vi "UNITEST MAIN v2.0.vi"() -> ()   [LabVIEW 2025] (continued)
        n1667 = Unbundle By Name(w2745) -> ("Main Screen.STOP"=w2752:refnum<vi>)
        n1668 = Unbundle By Name(w2745) -> ("Main Home Screen.GUI"=w2761:refnum<vi>)
        n1669 = property on="Property Node" class="TabCtl (strict)"(reference=w2757, "Value"=T16."HOME") -> (reference out=w2759:refnum<vi>, error out=w2758:errorcluster)  [unwired: 1 in]
        n1670 = property on="Property Node" class="TabCtl (strict)"(reference=w2761, "Value"=T15."Setup") -> (reference out=w2763:refnum<vi>, error out=w2762:errorcluster)  [unwired: 1 in]
        n1671 = property on="Property Node" class="Bool (strict)"(reference=w2753, "Visible"=TRUE ("Value"), "Value"=FALSE) -> (reference out=w2748:refnum<vi>, error out=w2754:errorcluster)  [unwired: 1 in]
        n1672 = property on="Property Node" class="Bool (strict)"(reference=w2752, "Value"=w2750, "Visible"=w2750) -> (reference out=w2747:refnum<vi>, error out=w2751:errorcluster)  [unwired: 1 in]
        n1673 = Close Reference(reference=w2763, error in (no error)=w2762) -> ()  [unwired: 1 out]
        n1674 = Close Reference(reference=w2759, error in (no error)=w2758) -> ()  [unwired: 1 out]
        n1675 = Close Reference(reference=w2748, error in (no error)=w2754) -> ()  [unwired: 1 out]
        n1676 = Close Reference(reference=w2747, error in (no error)=w2751) -> ()  [unwired: 1 out]
        n1677 = call "Reinitial Parameter After Test.vi"("error in (no error)"=w2765, "main ref"=w2745) -> ("error out"=w2746:errorcluster)  [unwired: 9 in]
      }
      frame "Start Test" {
        n1678 = Unbundle By Name(w2771) -> ("Environmental control.Acoustic Emission 3"=w2777:refnum<vi>)
        n1679 = property on="Property Node" class="Bool (strict)"(reference=w2777) -> (reference out=w2775:refnum<vi>, error out=w2776:errorcluster, "Value"=w2774:bool)  [unwired: 1 in]
        n1680 = Close Reference(reference=w2775, error in (no error)=w2776) -> ()  [unwired: 1 out]
        n1681 = case shown="True" w2774 {
          tunnel: w2773 -> [w2779 w2783]
          tunnel: [w2779 w2780] -> w2772
          tunnel: w2771 -> [_ w2781]
          frame False {
          }
          frame True {
            n1682 = call "Acq start.vi"("error in (no error)"=w2783, "Data Cluster"=w2781) -> ("error out"=w2782:errorcluster)  [unwired: 9 in]
            n1683 = call <vilib>:"Clear Errors.vi"("error in (no error)"=w2782) -> ("error out"=w2780:errorcluster)  [unwired: 5 in, 1 out]
          }
        }
        n1684 = call "Test Start Sequence.vi"("error in (no error)"=w2772, "Data Cluster"=w2771) -> ("error out"=w2778:errorcluster)  [unwired: 9 in]
      }
      frame "STOP" {
        n1685 = call "Test Stop.vi"("error in (no error)"=w2805, "Data Cluster"=w2784) -> ("error out"=w2785:errorcluster)  [unwired: 9 in]
        n1686 = Unbundle By Name(w2784) -> ("Main Screen.Load En"=w2804:refnum<vi>)
        n1687 = Unbundle By Name(w2784) -> ("Main Screen.CZ FF"=w2799:refnum<vi>)
        n1688 = Unbundle By Name(w2784) -> ("Main Screen.zFF"=w2796:refnum<vi>)
        n1689 = property on="Property Node" class="Bool (strict)"(reference=w2804, "DisabledEnum"=T31."Disabled and Grayed Out" ("Disabled")) -> (reference out=w2792:refnum<vi>, error out=w2803:errorcluster)  [unwired: 1 in]
        n1690 = property on="Property Node" class="Bool (strict)"(reference=w2799, "DisabledEnum"=T31."Disabled and Grayed Out" ("Disabled"), "Value"=FALSE ("Visible")) -> (reference out=w2798:refnum<vi>, error out=w2800:errorcluster)  [unwired: 1 in]
        n1691 = property on="Property Node" class="Bool (strict)"(reference=w2796, "DisabledEnum"=T31."Disabled and Grayed Out" ("Disabled"), "Value"=FALSE ("Visible")) -> (reference out=w2797:refnum<vi>, error out=w2795:errorcluster)  [unwired: 1 in]
        n1692 = Close Reference(reference=w2792, error in (no error)=w2803) -> ()  [unwired: 1 out]
        n1693 = Close Reference(reference=w2798, error in (no error)=w2800) -> ()  [unwired: 1 out]
        n1694 = Close Reference(reference=w2797, error in (no error)=w2795) -> ()  [unwired: 1 out]
        n1695 = Unbundle By Name(w2784) -> ("Environmental control.Acoustic Emission 3"=w2790:refnum<vi>)
        n1696 = property on="Property Node" class="Bool (strict)"(reference=w2790) -> (reference out=w2788:refnum<vi>, error out=w2789:errorcluster, "Value"=w2787:bool)  [unwired: 1 in]
        n1697 = Close Reference(reference=w2788, error in (no error)=w2789) -> ()  [unwired: 1 out]
        n1698 = case shown="False" w2787 {
          tunnel: w2785 -> [w2806 w2810]
          tunnel: [w2806 w2807] -> w2786
          tunnel: w2784 -> [_ w2808]
          frame False {
          }
          frame True {
            n1699 = call "Acq stop.vi"("error in (no error)"=w2810, "Data Cluster"=w2808) -> ("error out"=w2809:errorcluster)  [unwired: 9 in]
            n1700 = call <vilib>:"Clear Errors.vi"("error in (no error)"=w2809) -> ("error out"=w2807:errorcluster)  [unwired: 5 in, 1 out]
          }
        }
      }
      frame "PlaceModule" {
        n1701 = call "Place Module.vi"("error in (no error)"=w2813, "main ref"=w2811) -> ("error out"=w2812:errorcluster)  [unwired: 9 in]
      }
      frame "Stage Homing" {
        n1702 = call "HOMINING.vi"("error in (no error)"=w2816, "main ref"=w2814) -> ("error out"=w2815:errorcluster)  [unwired: 9 in]
      }
      frame "Clear 3" {
        n1703 = Unbundle By Name(w2818) -> ("Loading.Stribeck Table  For loading"=w2828:refnum<vi>)
        n1704 = Unbundle By Name(w2818) -> ("Loading.Clear 3"=w2819:refnum<vi>)
        n1705 = property on="Property Node" class="Bool (strict)"(reference=w2819, "Value"=FALSE) -> (reference out=w2821:refnum<vi>, error out=w2820:errorcluster)  [unwired: 1 in]
        n1706 = call "DATA ENCRYPT STRING FILE WRITE.vi"("error in (no error)"=w2824, "User Action"="User Pressed Clear  on Step Load Sequence", "main ref"=w2818) -> ("error out"=w2823:errorcluster)  [unwired: 6 in, 1 out]
        n1707 = property on="Property Node" class="Tbl (strict)"(reference=w2828, "Value"=string[][] []) -> (reference out=w2826:refnum<vi>, error out=w2827:errorcluster)  [unwired: 1 in]
        n1708 = Close Reference(reference=w2821, error in (no error)=w2820) -> ()  [unwired: 1 out]
        n1709 = Close Reference(reference=w2826, error in (no error)=w2827) -> ()  [unwired: 1 out]
      }
      frame "Set WTD" {
        n1710 = Unbundle By Name(w2829) -> ("Motion Module.Set WTD"=w2832:refnum<vi>)
        n1711 = property on="Property Node" class="Bool (strict)"(reference=w2832, "Value"=FALSE) -> (reference out=w2834:refnum<vi>, error out=w2833:errorcluster)  [unwired: 1 in]
        n1712 = call "DATA ENCRYPT STRING FILE WRITE.vi"("error in (no error)"=w2836, "User Action"="User Pressed  on Set Wear Track", "main ref"=w2829) -> ("error out"=w2835:errorcluster)  [unwired: 6 in, 1 out]
        n1713 = call "Sway wear trac set.vi"("error in (no error)"=w2835, "main ref"=w2829) -> ("error out"=w2830:errorcluster)  [unwired: 9 in]
        n1714 = Close Reference(reference=w2834, error in (no error)=w2833) -> ()  [unwired: 1 out]
      }
      frame "Import 2" {
        n1715 = call "File Dialog"("start path"=path "C:/LAB-IQ 150/User Defined Protocol", "error in"=w2845) -> ("selected path"=w2839:path, "cancelled"=w2842:bool, "error out"=w2844:errorcluster)  [unwired: 10 in, 1 out]
        n1716 = call <vilib>:"Clear Errors.vi"("error in (no error)"=w2844) -> ("error out"=w2841:errorcluster)  [unwired: 5 in, 1 out]
        n1717 = case shown="False" w2842 {
          tunnel: w2841 -> [w2855 w2856]
          tunnel: [w2847 w2856] -> w2840
          tunnel: w2839 -> [w2854 _]
          tunnel: w2838 -> [w2849 _]
          frame False {
            n1718 = call-poly <vilib>:"Read Delimited Spreadsheet.vi"("file path (dialog if empty)"=w2854, "error in (no error)"=w2855, "delimiter (\\t)"=":" ("delimiter (\\t)")) -> ("all rows"=w2846:string[][], "error out"=w2848:errorcluster)  [unwired: 7 in, 4 out]
            n1719 = Unbundle By Name(w2849) -> ("Motion Module.StepTable For Speed"=w2852:refnum<vi>)
            n1720 = property on="Property Node" class="Tbl (strict)"(reference=w2852, error in=w2848, "Value"=w2846) -> (reference out=w2850:refnum<vi>, error out=w2851:errorcluster)
            n1721 = Close Reference(reference=w2850, error in (no error)=w2851) -> (error out=w2847:errorcluster)
          }
          frame True {
          }
        }
      }
      frame "Save 2" {
        n1722 = Unbundle By Name(w2860) -> ("Motion Module.StepTable For Speed"=w2875:refnum<vi>)
        n1723 = property on="Property Node" class="Tbl (strict)"(reference=w2875) -> (reference out=w2873:refnum<vi>, error out=w2874:errorcluster, "Value"=w2871:string[][])  [unwired: 1 in]
        n1724 = call "File Dialog2"("start path"=path "C:/LAB-IQ 150/User Defined Protocol", "error in"=w2865) -> ("selected path"=w2868:path, "error out"=w2867:errorcluster)  [unwired: 10 in, 2 out]
        n1725 = call <vilib>:"Clear Errors.vi"("error in (no error)"=w2867) -> ("error out"=w2866:errorcluster)  [unwired: 5 in, 1 out]
        n1726 = Close Reference(reference=w2873, error in (no error)=w2874) -> ()  [unwired: 1 out]
        n1727 = call-poly <vilib>:"Write Delimited Spreadsheet.vi"("file path (dialog if empty)"=w2868, "2D data"=w2871, "append to file? (new file:F)"=TRUE, "error in (no error)"=w2866, "delimiter (\\t)"=":" ("delimiter (\\t)")) -> ("error out"=w2864:errorcluster)  [unwired: 9 in, 1 out]
        n1728 = call <vilib>:"Clear Errors.vi"("error in (no error)"=w2864) -> ("error out"=w2859:errorcluster)  [unwired: 5 in, 1 out]
        n1729 = Unbundle By Name(w2860) -> ("Motion Module.Save 2"=w2861:refnum<vi>)
        n1730 = property on="Property Node" class="Bool (strict)"(reference=w2861, error in=w2859, "Value"=FALSE) -> (reference out=w2863:refnum<vi>, error out=w2862:errorcluster)
        n1731 = Close Reference(reference=w2863, error in (no error)=w2862) -> (error out=w2858:errorcluster)
      }
      frame "Calculate Rotary" {
        n1732 = call "STEP LOAD MM_SEC AND RPM CONVERSION.vi"("error in (no error)"=w2879, "Data Cluster"=w2877) -> ("error out"=w2878:errorcluster)  [unwired: 9 in]
        n1733 = local write "calculate rotary"(FALSE) -> ()
      }
      frame "Clear List" {
        n1734 = Unbundle By Name(w2881) -> ("Environmental control.Sensors Picked"=w2888:refnum<vi>)
        n1735 = Unbundle By Name(w2881) -> ("Environmental control.Clear List"=w2882:refnum<vi>)
        n1736 = property on="Property Node" class="Bool (strict)"(reference=w2882, "Value"=FALSE) -> (reference out=w2884:refnum<vi>, error out=w2883:errorcluster)  [unwired: 1 in]
        n1737 = property on="Property Node" class="Str"(reference=w2888, "Value"="") -> (reference out=w2886:refnum<vi>, error out=w2887:errorcluster)  [unwired: 1 in]
        n1738 = Close Reference(reference=w2884, error in (no error)=w2883) -> ()  [unwired: 1 out]
        n1739 = Close Reference(reference=w2886, error in (no error)=w2887) -> ()  [unwired: 1 out]
      }
      frame "ClrLog" {
        n1740 = Unbundle By Name(w2891) -> ("Main Screen.ClrLog"=w2892:refnum<vi>)
        n1741 = Unbundle By Name(w2891) -> ("Main Screen.Trip Log"=w2898:refnum<vi>)
        n1742 = property on="Property Node" class="Bool (strict)"(reference=w2892, "Value"=FALSE) -> (reference out=w2894:refnum<vi>, error out=w2893:errorcluster)  [unwired: 1 in]
        n1743 = property on="Property Node" class="Str"(reference=w2898, "Value"="") -> (reference out=w2896:refnum<vi>, error out=w2897:errorcluster)  [unwired: 1 in]
        n1744 = Close Reference(reference=w2894, error in (no error)=w2893) -> ()  [unwired: 1 out]
        n1745 = Close Reference(reference=w2896, error in (no error)=w2897) -> ()  [unwired: 1 out]
      }
      frame "Add to list" {
        n1746 = Unbundle By Name(w2900) -> ("Environmental control.Sensors Picked"=w2906:refnum<vi>)
        n1747 = property on="Property Node" class="Str"(reference=w2906, error in=w2901, "Value"="") -> (reference out=w2904:refnum<vi>, error out=w2905:errorcluster)
        n1748 = Close Reference(reference=w2904, error in (no error)=w2905) -> (error out=w2902:errorcluster)
        n1749 = call "Add  to List Loop.vi"("error in (no error)"=w2902, "Data Cluster"=w2900) -> ("error out"=w2908:errorcluster)  [unwired: 9 in]
        n1750 = Unbundle By Name(w2900) -> ("Environmental control.Add to list"=w2910:refnum<vi>)
        n1751 = property on="Property Node" class="Bool (strict)"(reference=w2910, error in=w2908, "Value"=FALSE) -> (reference out=w2912:refnum<vi>, error out=w2911:errorcluster)
        n1752 = Close Reference(reference=w2912, error in (no error)=w2911) -> (error out=w2907:errorcluster)
      }
      frame "Disable Axis Jog Soft Limits" {
        n1753 = call "DATA ENCRYPT STRING FILE WRITE.vi"("error in (no error)"=w2916, "User Action"="User Pressed Disable Axis Jog Soft Limits in Main Screen", "main ref"=w2914) -> ("error out"=w2915:errorcluster)  [unwired: 6 in, 1 out]
      }
      frame "Home Service" {
        n1754 = Unbundle By Name(w2918) -> ("Main Home Screen.MainPage"=w2924:refnum<vi>)
        n1755 = Unbundle By Name(w2918) -> ("Main Home Screen.GUI"=w2922:refnum<vi>)
        n1756 = local write "Home Service"(FALSE ("Home Service")) -> ()
        n1757 = property on="Property Node" class="TabCtl (strict)"(reference=w2924, "Value"=T16."HOME") -> (reference out=w2926:refnum<vi>, error out=w2925:errorcluster)  [unwired: 1 in]
        n1758 = property on="Property Node" class="TabCtl (strict)"(reference=w2922, "Value"=T15."Setup") -> (reference out=w2920:refnum<vi>, error out=w2921:errorcluster)  [unwired: 1 in]
        n1759 = Close Reference(reference=w2926, error in (no error)=w2925) -> ()  [unwired: 1 out]
        n1760 = Close Reference(reference=w2920, error in (no error)=w2921) -> ()  [unwired: 1 out]
        n1761 = call "DATA ENCRYPT STRING FILE WRITE.vi"("error in (no error)"=w2929, "User Action"="User Pressed Home Service from Service Screen", "main ref"=w2918) -> ("error out"=w2928:errorcluster)  [unwired: 6 in, 1 out]
      }
      frame "Analysis Home" {
        n1762 = Unbundle By Name(w2931) -> ("Main Screen.Main Screen Tab"=w2934:refnum<vi>)
        n1763 = Unbundle By Name(w2931) -> ("Main Home Screen.MainPage"=w2941:refnum<vi>)
        n1764 = Unbundle By Name(w2931) -> ("Main Home Screen.GUI"=w2939:refnum<vi>)
        n1765 = local write "Analysis Home new"(FALSE ("Analysis Home new")) -> ()
        n1766 = property on="Property Node" class="TabCtl (strict)"(reference=w2934, "Value"=T19."  Acquire  ") -> (reference out=w2932:refnum<vi>, error out=w2933:errorcluster)  [unwired: 1 in]
        n1767 = property on="Property Node" class="TabCtl (strict)"(reference=w2941, "Value"=T16."HOME") -> (reference out=w2943:refnum<vi>, error out=w2942:errorcluster)  [unwired: 1 in]
        n1768 = property on="Property Node" class="TabCtl (strict)"(reference=w2939, "Value"=T15."Setup") -> (reference out=w2937:refnum<vi>, error out=w2938:errorcluster)  [unwired: 1 in]
        n1769 = Close Reference(reference=w2932, error in (no error)=w2933) -> ()  [unwired: 1 out]
        n1770 = Close Reference(reference=w2943, error in (no error)=w2942) -> ()  [unwired: 1 out]
        n1771 = Close Reference(reference=w2937, error in (no error)=w2938) -> ()  [unwired: 1 out]
        n1772 = call "DATA ENCRYPT STRING FILE WRITE.vi"("error in (no error)"=w2946, "User Action"="User Pressed Home from AnalysisScreen", "main ref"=w2931) -> ("error out"=w2945:errorcluster)  [unwired: 6 in, 1 out]
      }
      frame "Post Analysis" {
        n1773 = Unbundle By Name(w2949) -> ("Main Screen.Main Screen Tab"=w2952:refnum<vi>)
        n1774 = Unbundle By Name(w2949) -> ("Main Home Screen.MainPage"=w2958:refnum<vi>)
        n1775 = Unbundle By Name(w2949) -> ("Main Home Screen.GUI"=w2956:refnum<vi>)
        n1776 = property on="Property Node" class="TabCtl (strict)"(reference=w2952, "Value"=T19."Compare Files Rot") -> (reference out=w2950:refnum<vi>, error out=w2951:errorcluster)  [unwired: 1 in]
        n1777 = property on="Property Node" class="TabCtl (strict)"(reference=w2958, "Value"=T16."HOME") -> (reference out=w2960:refnum<vi>, error out=w2959:errorcluster)  [unwired: 1 in]
        n1778 = property on="Property Node" class="TabCtl (strict)"(reference=w2956, "Value"=T15."Begin") -> (reference out=w2954:refnum<vi>, error out=w2955:errorcluster)  [unwired: 1 in]
        n1779 = local write "Post Analysis"(FALSE ("Post Analysis")) -> ()
        n1780 = Close Reference(reference=w2950, error in (no error)=w2951) -> ()  [unwired: 1 out]
        n1781 = Close Reference(reference=w2960, error in (no error)=w2959) -> ()  [unwired: 1 out]
        n1782 = Close Reference(reference=w2954, error in (no error)=w2955) -> ()  [unwired: 1 out]
        n1783 = call "DATA ENCRYPT STRING FILE WRITE.vi"("error in (no error)"=w2963, "User Action"="User Pressed Post Analysis ", "main ref"=w2949) -> ("error out"=w2962:errorcluster)  [unwired: 6 in, 1 out]
      }
      frame "Edit Gain Constants" {
        n1784 = Unbundle By Name(w2965) -> ("About Screen.Heave and Surge COM Port:"=w2995:refnum<vi>)
        n1785 = Unbundle By Name(w2965) -> ("About Screen.Edit Gain Constants"=w2975:refnum<vi>)
        n1786 = Unbundle By Name(w2965) -> ("About Screen.Sway COM Port:"=w2992:refnum<vi>)
        n1787 = Unbundle By Name(w2965) -> ("About Screen.Ramp Port:"=w2969:refnum<vi>)
        n1788 = Unbundle By Name(w2965) -> ("About Screen.Temp Modbus:"=w2989:refnum<vi>)
        n1789 = Unbundle By Name(w2965) -> ("About Screen.Humidity Port:"=w2988:refnum<vi>)
        n1790 = Unbundle By Name(w2965) -> ("About Screen.Password"=w2983:refnum<vi>)
        n1791 = Unbundle By Name(w2965) -> ("About Screen.ECR Port:"=w2968:refnum<vi>)
        n1792 = property on="Property Node" class="VISAName"(reference=w2969, "DisabledEnum"=T31."Enabled" ("Disabled")) -> (reference out=w2971:refnum<vi>, error out=w2970:errorcluster)  [unwired: 1 in]
        n1793 = property on="Property Node" class="Bool (strict)"(reference=w2975, "Value"=FALSE) -> (reference out=w2976:refnum<vi>, error out=w2974:errorcluster)  [unwired: 1 in]
        n1794 = property on="Property Node" class="VISAName"(reference=w2968, "DisabledEnum"=T31."Enabled" ("Disabled")) -> (reference out=w2964:refnum<vi>, error out=w2967:errorcluster)  [unwired: 1 in]
        n1795 = property on="Property Node" class="VISAName"(reference=w2995, "DisabledEnum"=T31."Enabled" ("Disabled")) -> (reference out=w2996:refnum<vi>, error out=w2994:errorcluster)  [unwired: 1 in]
        n1796 = property on="Property Node" class="VISAName"(reference=w2992, "DisabledEnum"=T31."Enabled" ("Disabled")) -> (reference out=w2993:refnum<vi>, error out=w2991:errorcluster)  [unwired: 1 in]
        n1797 = property on="Property Node" class="VISAName"(reference=w2989, "DisabledEnum"=T31."Enabled" ("Disabled")) -> (reference out=w2977:refnum<vi>, error out=w2990:errorcluster)  [unwired: 1 in]
        n1798 = property on="Property Node" class="VISAName"(reference=w2988, "DisabledEnum"=T31."Enabled" ("Disabled")) -> (reference out=w2986:refnum<vi>, error out=w2987:errorcluster)  [unwired: 1 in]
        n1799 = property on="Property Node" class="Str"(reference=w2983, "Visible"=FALSE) -> (reference out=w2985:refnum<vi>, error out=w2984:errorcluster)  [unwired: 1 in]
        n1800 = Close Reference(reference=w2971, error in (no error)=w2970) -> ()  [unwired: 1 out]
        n1801 = Close Reference(reference=w2985, error in (no error)=w2984) -> ()  [unwired: 1 out]
        n1802 = Close Reference(reference=w2964, error in (no error)=w2967) -> ()  [unwired: 1 out]
        n1803 = Close Reference(reference=w2976, error in (no error)=w2974) -> ()  [unwired: 1 out]
        n1804 = Close Reference(reference=w2996, error in (no error)=w2994) -> ()  [unwired: 1 out]
        n1805 = Close Reference(reference=w2993, error in (no error)=w2991) -> ()  [unwired: 1 out]
        n1806 = Close Reference(reference=w2977, error in (no error)=w2990) -> ()  [unwired: 1 out]
        n1807 = Close Reference(reference=w2986, error in (no error)=w2987) -> ()  [unwired: 1 out]
        n1808 = call "DATA ENCRYPT STRING FILE WRITE.vi"("error in (no error)"=w2999, "User Action"="User Pressed Home Service from Service Screen", "main ref"=w2965) -> ("error out"=w2998:errorcluster)  [unwired: 6 in, 1 out]
      }
      frame "Advanced Setting" {
        n1809 = Unbundle By Name(w3001) -> ("About Screen.Advanced Setting"=w3003:refnum<vi>)
        n1810 = property on="Property Node" class="Bool (strict)"(reference=w3003) -> (reference out=w3004:refnum<vi>, error out=w3002:errorcluster, "Value"=w3000:bool)  [unwired: 1 in]
        n1811 = Close Reference(reference=w3004, error in (no error)=w3002) -> ()  [unwired: 1 out]
        n1812 = case shown="True" w3000 {
          tunnel: w3001 -> [w3009 w3034]
          frame True {
            n1813 = Unbundle By Name(w3009) -> ("About Screen.Heave and Surge COM Port:"=w3031:refnum<vi>)
            n1814 = Unbundle By Name(w3009) -> ("About Screen.Edit Gain Constants"=w3011:refnum<vi>)
            n1815 = Unbundle By Name(w3009) -> ("About Screen.Sway COM Port:"=w3028:refnum<vi>)
            n1816 = Unbundle By Name(w3009) -> ("About Screen.Temp Modbus:"=w3025:refnum<vi>)
            n1817 = Unbundle By Name(w3009) -> ("About Screen.Humidity Port:"=w3024:refnum<vi>)
            n1818 = Unbundle By Name(w3009) -> ("About Screen.Password"=w3019:refnum<vi>)
            n1819 = property on="Property Node" class="Bool (strict)"(reference=w3011, "Value"=FALSE) -> (reference out=w3012:refnum<vi>, error out=w3010:errorcluster)  [unwired: 1 in]
            n1820 = property on="Property Node" class="VISAName"(reference=w3031, "DisabledEnum"=T31."Disabled and Grayed Out" ("Disabled")) -> (reference out=w3032:refnum<vi>, error out=w3030:errorcluster)  [unwired: 1 in]
            n1821 = property on="Property Node" class="VISAName"(reference=w3028, "DisabledEnum"=T31."Disabled and Grayed Out" ("Disabled")) -> (reference out=w3029:refnum<vi>, error out=w3027:errorcluster)  [unwired: 1 in]
            n1822 = property on="Property Node" class="VISAName"(reference=w3025, "DisabledEnum"=T31."Disabled and Grayed Out" ("Disabled")) -> (reference out=w3013:refnum<vi>, error out=w3026:errorcluster)  [unwired: 1 in]
            n1823 = property on="Property Node" class="VISAName"(reference=w3024, "DisabledEnum"=T31."Disabled and Grayed Out" ("Disabled")) -> (reference out=w3022:refnum<vi>, error out=w3023:errorcluster)  [unwired: 1 in]
            n1824 = property on="Property Node" class="Str"(reference=w3019, "Visible"=TRUE) -> (reference out=w3021:refnum<vi>, error out=w3020:errorcluster)  [unwired: 1 in]
            n1825 = Close Reference(reference=w3012, error in (no error)=w3010) -> ()  [unwired: 1 out]
            n1826 = Close Reference(reference=w3032, error in (no error)=w3030) -> ()  [unwired: 1 out]
            n1827 = Close Reference(reference=w3029, error in (no error)=w3027) -> ()  [unwired: 1 out]
            n1828 = Close Reference(reference=w3013, error in (no error)=w3026) -> ()  [unwired: 1 out]
            n1829 = Close Reference(reference=w3022, error in (no error)=w3023) -> ()  [unwired: 1 out]
            n1830 = Close Reference(reference=w3021, error in (no error)=w3020) -> ()  [unwired: 1 out]
          }
          frame False {
            n1831 = Unbundle By Name(w3034) -> ("About Screen.Heave and Surge COM Port:"=w3056:refnum<vi>)
            n1832 = Unbundle By Name(w3034) -> ("About Screen.Edit Gain Constants"=w3036:refnum<vi>)
            n1833 = Unbundle By Name(w3034) -> ("About Screen.Sway COM Port:"=w3053:refnum<vi>)
            n1834 = Unbundle By Name(w3034) -> ("About Screen.Temp Modbus:"=w3050:refnum<vi>)
            n1835 = Unbundle By Name(w3034) -> ("About Screen.Humidity Port:"=w3049:refnum<vi>)
            n1836 = Unbundle By Name(w3034) -> ("About Screen.Password"=w3044:refnum<vi>)
            n1837 = property on="Property Node" class="Bool (strict)"(reference=w3036, "Value"=FALSE) -> (reference out=w3037:refnum<vi>, error out=w3035:errorcluster)  [unwired: 1 in]
            n1838 = property on="Property Node" class="VISAName"(reference=w3056, "DisabledEnum"=T31."Disabled and Grayed Out" ("Disabled")) -> (reference out=w3057:refnum<vi>, error out=w3055:errorcluster)  [unwired: 1 in]
            n1839 = property on="Property Node" class="VISAName"(reference=w3053, "DisabledEnum"=T31."Disabled and Grayed Out" ("Disabled")) -> (reference out=w3054:refnum<vi>, error out=w3052:errorcluster)  [unwired: 1 in]
            n1840 = property on="Property Node" class="VISAName"(reference=w3050, "DisabledEnum"=T31."Disabled and Grayed Out" ("Disabled")) -> (reference out=w3038:refnum<vi>, error out=w3051:errorcluster)  [unwired: 1 in]
            n1841 = property on="Property Node" class="VISAName"(reference=w3049, "DisabledEnum"=T31."Disabled and Grayed Out" ("Disabled")) -> (reference out=w3047:refnum<vi>, error out=w3048:errorcluster)  [unwired: 1 in]
            n1842 = property on="Property Node" class="Str"(reference=w3044, "Visible"=FALSE) -> (reference out=w3046:refnum<vi>, error out=w3045:errorcluster)  [unwired: 1 in]
            n1843 = Close Reference(reference=w3037, error in (no error)=w3035) -> ()  [unwired: 1 out]
            n1844 = Close Reference(reference=w3057, error in (no error)=w3055) -> ()  [unwired: 1 out]
            n1845 = Close Reference(reference=w3054, error in (no error)=w3052) -> ()  [unwired: 1 out]
            n1846 = Close Reference(reference=w3038, error in (no error)=w3051) -> ()  [unwired: 1 out]
            n1847 = Close Reference(reference=w3047, error in (no error)=w3048) -> ()  [unwired: 1 out]
            n1848 = Close Reference(reference=w3046, error in (no error)=w3045) -> ()  [unwired: 1 out]
          }
        }
        n1849 = call "DATA ENCRYPT STRING FILE WRITE.vi"("error in (no error)"=w3007, "User Action"="User Pressed Advance Setting in Service Screen", "main ref"=w3001) -> ("error out"=w3006:errorcluster)  [unwired: 6 in, 1 out]
      }
      frame "Password" {
        n1850 = Unbundle By Name(w3058) -> ("About Screen.Password"=w3064:refnum<vi>)
        n1851 = property on="Property Node" class="Str"(reference=w3064) -> (reference out=w3065:refnum<vi>, error out=w3063:errorcluster, "Value"=w3062:string)  [unwired: 1 in]
        n1852 = call <vilib>:"Trim Whitespace.vi"("string"=w3062) -> ("trimmed string"=w3061:string)  [unwired: 1 in]
        n1853 = Close Reference(reference=w3065, error in (no error)=w3063) -> ()  [unwired: 1 out]
        n1854 = Equal?(x=w3061, y="UT150$") -> (x = y?=w3059:bool)
        n1855 = case shown="True" w3059 {
          tunnel: w3058 -> [_ w3068]
          frame False {
          }
          frame True {
            n1856 = Unbundle By Name(w3068) -> ("Main Screen.Main Screen Tab"=w3070:refnum<vi>)
            n1857 = Unbundle By Name(w3068) -> ("Main Home Screen.GUI"=w3074:refnum<vi>)
            n1858 = Unbundle By Name(w3068) -> ("About Screen.Password"=w3078:refnum<vi>)
            n1859 = property on="Property Node" class="TabCtl (strict)"(reference=w3074, "Value"=T15."Begin") -> (reference out=w3075:refnum<vi>, error out=w3073:errorcluster)  [unwired: 1 in]
            n1860 = property on="Property Node" class="TabCtl (strict)"(reference=w3070, "Value"=T19."Service") -> (reference out=w3069:refnum<vi>, error out=w3071:errorcluster)  [unwired: 1 in]
            n1861 = property on="Property Node" class="Str"(reference=w3078, "Value"="") -> (reference out=w3079:refnum<vi>, error out=w3077:errorcluster)  [unwired: 1 in]
            n1862 = Close Reference(reference=w3079, error in (no error)=w3077) -> ()  [unwired: 1 out]
            n1863 = Close Reference(reference=w3075, error in (no error)=w3073) -> ()  [unwired: 1 out]
            n1864 = Close Reference(reference=w3069, error in (no error)=w3071) -> ()  [unwired: 1 out]
          }
        }
      }
      frame "Service About" {
        n1865 = Unbundle By Name(w3081) -> ("Main Screen.Main Screen Tab"=w3084:refnum<vi>)
        n1866 = Unbundle By Name(w3081) -> ("Main Home Screen.GUI"=w3088:refnum<vi>)
        n1867 = local write "Service About"(FALSE ("Service About")) -> ()
        n1868 = property on="Property Node" class="TabCtl (strict)"(reference=w3088, "Value"=T15."Begin") -> (reference out=w3089:refnum<vi>, error out=w3087:errorcluster)  [unwired: 1 in]
        n1869 = property on="Property Node" class="TabCtl (strict)"(reference=w3084, "Value"=T19."About") -> (reference out=w3083:refnum<vi>, error out=w3085:errorcluster)  [unwired: 1 in]
        n1870 = Close Reference(reference=w3089, error in (no error)=w3087) -> ()  [unwired: 1 out]
        n1871 = Close Reference(reference=w3083, error in (no error)=w3085) -> ()  [unwired: 1 out]
      }
      frame "OPEN 1" {
        n1872 = Unbundle By Name(w3093) -> ("Analysis Screen.File 1 Discription"=w3102:refnum<vi>)
        n1873 = property on="Property Node" class="Str"(reference=w3102, error in=w3100, "Value"="") -> (reference out=w3103:refnum<vi>, error out=w3101:errorcluster)
        n1874 = Close Reference(reference=w3103, error in (no error)=w3101) -> (error out=w3099:errorcluster)
        n1875 = call <vilib>:"Application Directory.vi"() -> ("Application Directory"=w3107:path)
        n1876 = Unbundle By Name(w3093) -> ("Analysis Screen.OPEN 1"=w3095:refnum<vi>)
        n1877 = Build Path(base path=w3107, name or relative path="data") -> (appended path=w3105:path)
        n1878 = property on="Property Node" class="Bool (strict)"(reference=w3095, "Value"=FALSE) -> (reference out=w3096:refnum<vi>, error out=w3094:errorcluster)  [unwired: 1 in]
        n1879 = call "File Dialog3"("start path"=w3105, "error in"=w3099) -> ("selected path"=w3104:path, "cancelled"=w3091:bool, "error out"=w3108:errorcluster)  [unwired: 10 in, 1 out]
        n1880 = case shown="True" w3091 {
          tunnel: w3108 -> [w3122 _]
          tunnel: w3104 -> [w3118 _]
          tunnel: [w3110 _] -> w3097
          tunnel: w3093 -> [w3109 w3124]
          frame False {
            n1881 = Path To String(path=w3118) -> (string=w3117:string)
            n1882 = Unbundle By Name(w3109) -> ("Analysis Screen.File Name 1"=w3120:refnum<vi>)
            n1883 = call <vilib>:"Clear Errors.vi"("error in (no error)"=w3122) -> ("error out"=w3116:errorcluster)  [unwired: 5 in, 1 out]
            n1884 = property on="Property Node" class="Str"(reference=w3120, "Value"=w3117) -> (reference out=w3121:refnum<vi>, error out=w3119:errorcluster)  [unwired: 1 in]
            n1885 = call "INI FILE READ.vi"("error in (no error)"=w3116, "File Path"=w3117) -> ("error out"=w3112:errorcluster, "concatenated string"=w3111:string)  [unwired: 8 in]
            n1886 = Unbundle By Name(w3109) -> ("Analysis Screen.File 1 Discription"=w3114:refnum<vi>)
            n1887 = Close Reference(reference=w3121, error in (no error)=w3119) -> ()  [unwired: 1 out]
            n1888 = property on="Property Node" class="Str"(reference=w3114, error in=w3112, "Value"=w3111) -> (reference out=w3115:refnum<vi>, error out=w3113:errorcluster)
            n1889 = Close Reference(reference=w3115, error in (no error)=w3113) -> (error out=w3110:errorcluster)
          }
          frame True {
            n1890 = Unbundle By Name(w3124) -> ("Analysis Screen.File 1 Discription"=w3126:refnum<vi>)
            n1891 = Unbundle By Name(w3124) -> ("Analysis Screen.File Name 1"=w3130:refnum<vi>)
            n1892 = property on="Property Node" class="Str"(reference=w3126, "Value"="") -> (reference out=w3127:refnum<vi>, error out=w3125:errorcluster)  [unwired: 1 in]
            n1893 = property on="Property Node" class="Str"(reference=w3130, "Value"="") -> (reference out=w3131:refnum<vi>, error out=w3129:errorcluster)  [unwired: 1 in]
            n1894 = Close Reference(reference=w3127, error in (no error)=w3125) -> ()  [unwired: 1 out]
            n1895 = Close Reference(reference=w3131, error in (no error)=w3129) -> ()  [unwired: 1 out]
          }
        }
        n1896 = Close Reference(reference=w3096, error in (no error)=w3094) -> ()  [unwired: 1 out]
      }
      frame "OPEN 2" {
        n1897 = Unbundle By Name(w3134) -> ("Analysis Screen.File 2 Discription"=w3143:refnum<vi>)
        n1898 = property on="Property Node" class="Str"(reference=w3143, error in=w3141, "Value"="") -> (reference out=w3144:refnum<vi>, error out=w3142:errorcluster)
        n1899 = Close Reference(reference=w3144, error in (no error)=w3142) -> (error out=w3140:errorcluster)
        n1900 = call <vilib>:"Application Directory.vi"() -> ("Application Directory"=w3148:path)
        n1901 = Unbundle By Name(w3134) -> ("Analysis Screen.OPEN 2"=w3136:refnum<vi>)
        n1902 = Build Path(base path=w3148, name or relative path="data") -> (appended path=w3146:path)
        n1903 = property on="Property Node" class="Bool (strict)"(reference=w3136, "Value"=FALSE) -> (reference out=w3137:refnum<vi>, error out=w3135:errorcluster)  [unwired: 1 in]
        n1904 = call "File Dialog4"("start path"=w3146, "error in"=w3140) -> ("selected path"=w3145:path, "cancelled"=w3132:bool, "error out"=w3149:errorcluster)  [unwired: 10 in, 1 out]
        n1905 = case shown="True" w3132 {
          tunnel: w3149 -> [w3163 w3165]
          tunnel: w3145 -> [w3159 _]
          tunnel: [w3151 w3164] -> w3138
          tunnel: w3134 -> [w3150 w3167]
          frame False {
            n1906 = Path To String(path=w3159) -> (string=w3158:string)
            n1907 = Unbundle By Name(w3150) -> ("Analysis Screen.File Name 2"=w3161:refnum<vi>)
            n1908 = call <vilib>:"Clear Errors.vi"("error in (no error)"=w3163) -> ("error out"=w3157:errorcluster)  [unwired: 5 in, 1 out]
            n1909 = property on="Property Node" class="Str"(reference=w3161, "Value"=w3158) -> (reference out=w3162:refnum<vi>, error out=w3160:errorcluster)  [unwired: 1 in]
            n1910 = call "INI FILE READ.vi"("error in (no error)"=w3157, "File Path"=w3158) -> ("error out"=w3153:errorcluster, "concatenated string"=w3152:string)  [unwired: 8 in]
            n1911 = Unbundle By Name(w3150) -> ("Analysis Screen.File 2 Discription"=w3155:refnum<vi>)
            n1912 = Close Reference(reference=w3162, error in (no error)=w3160) -> ()  [unwired: 1 out]
            n1913 = property on="Property Node" class="Str"(reference=w3155, error in=w3153, "Value"=w3152) -> (reference out=w3156:refnum<vi>, error out=w3154:errorcluster)
            n1914 = Close Reference(reference=w3156, error in (no error)=w3154) -> (error out=w3151:errorcluster)
          }
          frame True {
            n1915 = Unbundle By Name(w3167) -> ("Analysis Screen.File Name 2"=w3173:refnum<vi>)
            n1916 = Unbundle By Name(w3167) -> ("Analysis Screen.File 2 Discription"=w3169:refnum<vi>)
            n1917 = property on="Property Node" class="Str"(reference=w3173, "Value"="") -> (reference out=w3174:refnum<vi>, error out=w3172:errorcluster)  [unwired: 1 in]
            n1918 = property on="Property Node" class="Str"(reference=w3169, "Value"="") -> (reference out=w3168:refnum<vi>, error out=w3170:errorcluster)  [unwired: 1 in]
            n1919 = call <vilib>:"Clear Errors.vi"("error in (no error)"=w3165) -> ("error out"=w3164:errorcluster)  [unwired: 5 in, 1 out]
            n1920 = Close Reference(reference=w3168, error in (no error)=w3170) -> ()  [unwired: 1 out]
            n1921 = Close Reference(reference=w3174, error in (no error)=w3172) -> ()  [unwired: 1 out]
          }
        }
        n1922 = Close Reference(reference=w3137, error in (no error)=w3135) -> ()  [unwired: 1 out]
      }
      frame "OPEN 3" {
        # "3416\n4017\n4554"
        n1923 = Unbundle By Name(w3177) -> ("Analysis Screen.File 3 Discription"=w3186:refnum<vi>)
        n1924 = property on="Property Node" class="Str"(reference=w3186, error in=w3184, "Value"="") -> (reference out=w3187:refnum<vi>, error out=w3185:errorcluster)
        n1925 = Close Reference(reference=w3187, error in (no error)=w3185) -> (error out=w3183:errorcluster)
        n1926 = call <vilib>:"Application Directory.vi"() -> ("Application Directory"=w3191:path)
        n1927 = Unbundle By Name(w3177) -> ("Analysis Screen.OPEN 3"=w3179:refnum<vi>)
        n1928 = Build Path(base path=w3191, name or relative path="data") -> (appended path=w3189:path)
        n1929 = property on="Property Node" class="Bool (strict)"(reference=w3179, "Value"=FALSE) -> (reference out=w3180:refnum<vi>, error out=w3178:errorcluster)  [unwired: 1 in]
        n1930 = call "File Dialog5"("start path"=w3189, "error in"=w3183) -> ("selected path"=w3188:path, "cancelled"=w3175:bool, "error out"=w3192:errorcluster)  [unwired: 10 in, 1 out]
        n1931 = case shown="True" w3175 {
          tunnel: w3192 -> [w3206 w3208]
          tunnel: w3188 -> [w3202 _]
          tunnel: [w3194 w3207] -> w3181
          tunnel: w3177 -> [w3193 w3210]
          frame False {
            n1932 = Path To String(path=w3202) -> (string=w3201:string)
            n1933 = Unbundle By Name(w3193) -> ("Analysis Screen.File Name 3"=w3204:refnum<vi>)
            n1934 = call <vilib>:"Clear Errors.vi"("error in (no error)"=w3206) -> ("error out"=w3200:errorcluster)  [unwired: 5 in, 1 out]
            n1935 = property on="Property Node" class="Str"(reference=w3204, "Value"=w3201) -> (reference out=w3205:refnum<vi>, error out=w3203:errorcluster)  [unwired: 1 in]
            n1936 = call "INI FILE READ.vi"("error in (no error)"=w3200, "File Path"=w3201) -> ("error out"=w3196:errorcluster, "concatenated string"=w3195:string)  [unwired: 8 in]
            n1937 = Unbundle By Name(w3193) -> ("Analysis Screen.File 3 Discription"=w3198:refnum<vi>)
            n1938 = Close Reference(reference=w3205, error in (no error)=w3203) -> ()  [unwired: 1 out]
            n1939 = property on="Property Node" class="Str"(reference=w3198, error in=w3196, "Value"=w3195) -> (reference out=w3199:refnum<vi>, error out=w3197:errorcluster)
            n1940 = Close Reference(reference=w3199, error in (no error)=w3197) -> (error out=w3194:errorcluster)
          }
          frame True {
            n1941 = Unbundle By Name(w3210) -> ("Analysis Screen.File Name 3"=w3216:refnum<vi>)
            n1942 = Unbundle By Name(w3210) -> ("Analysis Screen.File 3 Discription"=w3212:refnum<vi>)
            n1943 = property on="Property Node" class="Str"(reference=w3216, "Value"="") -> (reference out=w3217:refnum<vi>, error out=w3215:errorcluster)  [unwired: 1 in]
            n1944 = property on="Property Node" class="Str"(reference=w3212, "Value"="") -> (reference out=w3211:refnum<vi>, error out=w3213:errorcluster)  [unwired: 1 in]
            n1945 = Close Reference(reference=w3211, error in (no error)=w3213) -> ()  [unwired: 1 out]
            n1946 = Close Reference(reference=w3217, error in (no error)=w3215) -> ()  [unwired: 1 out]
            n1947 = call <vilib>:"Clear Errors.vi"("error in (no error)"=w3208) -> ("error out"=w3207:errorcluster)  [unwired: 5 in, 1 out]
          }
        }
        n1948 = Close Reference(reference=w3180, error in (no error)=w3178) -> ()  [unwired: 1 out]
      }
      frame "OPEN 4" {
        n1949 = Unbundle By Name(w3220) -> ("Analysis Screen.File 4 Discription"=w3229:refnum<vi>)
        n1950 = property on="Property Node" class="Str"(reference=w3229, error in=w3227, "Value"="") -> (reference out=w3230:refnum<vi>, error out=w3228:errorcluster)
        n1951 = Close Reference(reference=w3230, error in (no error)=w3228) -> (error out=w3226:errorcluster)
        n1952 = call <vilib>:"Application Directory.vi"() -> ("Application Directory"=w3234:path)
        n1953 = Unbundle By Name(w3220) -> ("Analysis Screen.OPEN 4"=w3222:refnum<vi>)
        n1954 = Build Path(base path=w3234, name or relative path="data") -> (appended path=w3232:path)
        n1955 = property on="Property Node" class="Bool (strict)"(reference=w3222, "Value"=FALSE) -> (reference out=w3223:refnum<vi>, error out=w3221:errorcluster)  [unwired: 1 in]
        n1956 = call "File Dialog6"("start path"=w3232, "error in"=w3226) -> ("selected path"=w3231:path, "cancelled"=w3218:bool, "error out"=w3235:errorcluster)  [unwired: 10 in, 1 out]
        n1957 = case shown="True" w3218 {
          tunnel: w3235 -> [w3249 w3251]
          tunnel: w3231 -> [w3245 _]
          tunnel: [w3237 w3250] -> w3224
          tunnel: w3220 -> [w3236 w3253]
          frame False {
            n1958 = Path To String(path=w3245) -> (string=w3244:string)
            n1959 = Unbundle By Name(w3236) -> ("Analysis Screen.File Name 4"=w3247:refnum<vi>)
            n1960 = call <vilib>:"Clear Errors.vi"("error in (no error)"=w3249) -> ("error out"=w3243:errorcluster)  [unwired: 5 in, 1 out]
            n1961 = property on="Property Node" class="Str"(reference=w3247, "Value"=w3244) -> (reference out=w3248:refnum<vi>, error out=w3246:errorcluster)  [unwired: 1 in]
            n1962 = call "INI FILE READ.vi"("error in (no error)"=w3243, "File Path"=w3244) -> ("error out"=w3239:errorcluster, "concatenated string"=w3238:string)  [unwired: 8 in]
            n1963 = Unbundle By Name(w3236) -> ("Analysis Screen.File 4 Discription"=w3241:refnum<vi>)
            n1964 = Close Reference(reference=w3248, error in (no error)=w3246) -> ()  [unwired: 1 out]
            n1965 = property on="Property Node" class="Str"(reference=w3241, error in=w3239, "Value"=w3238) -> (reference out=w3242:refnum<vi>, error out=w3240:errorcluster)
            n1966 = Close Reference(reference=w3242, error in (no error)=w3240) -> (error out=w3237:errorcluster)
          }
          frame True {
            n1967 = Unbundle By Name(w3253) -> ("Analysis Screen.File Name 4"=w3259:refnum<vi>)
            n1968 = Unbundle By Name(w3253) -> ("Analysis Screen.File 4 Discription"=w3255:refnum<vi>)
            n1969 = property on="Property Node" class="Str"(reference=w3259, "Value"="") -> (reference out=w3260:refnum<vi>, error out=w3258:errorcluster)  [unwired: 1 in]
            n1970 = property on="Property Node" class="Str"(reference=w3255, "Value"="") -> (reference out=w3254:refnum<vi>, error out=w3256:errorcluster)  [unwired: 1 in]
            n1971 = Close Reference(reference=w3254, error in (no error)=w3256) -> ()  [unwired: 1 out]
            n1972 = Close Reference(reference=w3260, error in (no error)=w3258) -> ()  [unwired: 1 out]
            n1973 = call <vilib>:"Clear Errors.vi"("error in (no error)"=w3251) -> ("error out"=w3250:errorcluster)  [unwired: 5 in, 1 out]
          }
        }
        n1974 = Close Reference(reference=w3223, error in (no error)=w3221) -> ()  [unwired: 1 out]
      }
      frame "Refresh 2" {
        n1975 = call "Data Log Refresh.vi"("error in (no error)"=w3263, "Data Cluster"=w3262) -> ("error out"=w3264:errorcluster)  [unwired: 9 in]
        n1976 = local write "Refresh 2"(FALSE ("Refresh 2")) -> ()
      }
      frame "Scratch Mode" {
        n1977 = Unbundle By Name(w3265) -> ("Motion Module.Scratch Mode"=w3268:refnum<vi>)
        n1978 = property on="Property Node" class="Ring (strict)"(reference=w3268) -> (reference out=w3269:refnum<vi>, error out=w3267:errorcluster, "Value"=w3266:u16)  [unwired: 1 in]
        n1979 = Close Reference(reference=w3269, error in (no error)=w3267) -> ()  [unwired: 1 out]
        n1980 = case shown="2" w3266 {
          tunnel: w3265 -> [w3272 w3276]
          frame 0, Default {
            n1981 = Unbundle By Name(w3272) -> ("Motion Module.No of Scratch"=w3274:refnum<vi>)
            n1982 = property on="Property Node" class="DigNum (strict)"(reference=w3274, "Visible"=FALSE) -> (reference out=w3275:refnum<vi>, error out=w3273:errorcluster)  [unwired: 1 in]
            n1983 = Close Reference(reference=w3275, error in (no error)=w3273) -> ()  [unwired: 1 out]
          }
          frame 2 {
            n1984 = Unbundle By Name(w3276) -> ("Motion Module.No of Scratch"=w3279:refnum<vi>)
            n1985 = property on="Property Node" class="DigNum (strict)"(reference=w3279, "Visible"=TRUE) -> (reference out=w3280:refnum<vi>, error out=w3278:errorcluster)  [unwired: 1 in]
            n1986 = Close Reference(reference=w3280, error in (no error)=w3278) -> ()  [unwired: 1 out]
          }
        }
      }
      frame "Export" {
        n1987 = call "Export file.vi"("error in (no error)"=w3289, "Data Cluster"=w3282) -> ("error out"=w3284:errorcluster)  [unwired: 9 in]
        n1988 = call "DATA ENCRYPT STRING FILE WRITE.vi"("error in (no error)"=w3284, "User Action"="User Pressed  Export ", "main ref"=w3282) -> ("error out"=w3283:errorcluster)  [unwired: 6 in, 1 out]
        n1989 = Unbundle By Name(w3282) -> ("Analysis Screen.Export"=w3287:refnum<vi>)
        n1990 = property on="Property Node" class="Bool (strict)"(reference=w3287, "Value"=FALSE) -> (reference out=w3288:refnum<vi>, error out=w3286:errorcluster)  [unwired: 1 in]
        n1991 = Close Reference(reference=w3288, error in (no error)=w3286) -> ()  [unwired: 1 out]
      }
      frame "Traction Receipe Update Details" {
